vi "test_PhotonPoseEstimator_pnpDistanceTrigSolve.vi"(8 "error in (no error)":errorcluster) -> (0 "error out":errorcluster, 3 "Test Passed":bool)   [LabVIEW 2019]
uses:
  <vilib>/Rock Robotics/WPI/ThirdParty/PhotonVisionLib/TypeDef/PhotonEstimatedRobotPoseType.ctl
  <vilib>/Rock Robotics/WPI/ThirdParty/JAS_Junk/TrajLib/TypeDef/POSE3D.ctl
  <vilib>/Rock Robotics/WPI/ThirdParty/JAS_Junk/TrajLib/TypeDef/TRANSLATION3D.ctl
  <vilib>/Rock Robotics/WPI/ThirdParty/JAS_Junk/TrajLib/TypeDef/ROTATION3D.ctl
  <vilib>/Rock Robotics/WPI/ThirdParty/JAS_Junk/TrajLib/TypeDef/QUATERNION.ctl
  <vilib>/Rock Robotics/WPI/ThirdParty/PhotonVisionLib/TypeDef/PhotonTrackedTargetType.ctl
  <vilib>/Rock Robotics/WPI/ThirdParty/PhotonVisionLib/TypeDef/TargetCornerType.ctl
  <vilib>/Rock Robotics/WPI/ThirdParty/JAS_Junk/TrajLib/TypeDef/TRANSFORM3D.ctl
  <vilib>/Rock Robotics/WPI/ThirdParty/PhotonVisionLib/Enum/PhotonPoseStrategy_ENUM.ctl
  <vilib>/Rock Robotics/WPI/ThirdParty/JAS_Junk/TrajLib/VI/Quaternion_New_Default.vi
  <vilib>/Rock Robotics/WPI/ThirdParty/JAS_Junk/TrajLib/VI/Quaternion_New.vi
  <vilib>/Rock Robotics/WPI/ThirdParty/PhotonVisionLib/SubVI/PhotonTargetModel_New_AprilTag36H11.vi
  <vilib>/Rock Robotics/WPI/ThirdParty/JAS_Junk/TrajLib/VI/TimeInterpRotation2d_New.vi
  <vilib>/Rock Robotics/WPI/ThirdParty/JAS_Junk/TrajLib/VI/TimeInterpRotation2d_AddSample.vi
  <vilib>/Rock Robotics/WPI/ThirdParty/JAS_Junk/TrajLib/VI/Rotation3d_ToRotation2d.vi
  <vilib>/Rock Robotics/WPI/ThirdParty/PhotonVisionLib/SubVI/PhotonPoseEstimator_Update_All.vi
  <vilib>/Rock Robotics/WPI/ThirdParty/JAS_Junk/TrajLib/VI/Quaternion_Get_All.vi
  <vilib>/Rock Robotics/WPI/ThirdParty/JAS_Junk/TrajLib/VI/Rotation3d_GetQuaterion.vi
  <vilib>/Rock Robotics/WPI/ThirdParty/PhotonVisionLib/SubVI/PhotonPoseEstimator_GetEmptyPose.vi
  <vilib>/Rock Robotics/WPI/ThirdParty/PhotonVisionLib/SubVI/PhotonPoseEstimator_EstimatePnpDistanceTrigSolvePose.vi
  <vilib>/Rock Robotics/WPI/ThirdParty/PhotonVisionLib/SubVI/PhotonPoseEstimator_SetLastPose.vi
  <vilib>/Rock Robotics/WPI/ThirdParty/JAS_Junk/TrajLib/VI/Transform3d_Equals.vi
  <vilib>/Rock Robotics/WPI/ThirdParty/PhotonVisionLib/SubVI/PhotonPoseEstimator_SetCamera.vi
  <vilib>/Rock Robotics/WPI/ThirdParty/PhotonVisionLib/SubVI/PhotonPoseEstimator_SetRobotToCameraTransform.vi
  <vilib>/Rock Robotics/WPI/ThirdParty/PhotonVisionLib/SubVI/PhotonEstimatedRobotPose_GetAll.vi
  <vilib>/Rock Robotics/WPI/ThirdParty/JAS_Junk/TrajLib/VI/Pose3d_ToPose2d.vi
  <vilib>/Rock Robotics/WPI/ThirdParty/PhotonVisionLib/SubVI/PhotonTargetModel_New_RectPlanar.vi
  <vilib>/Rock Robotics/WPI/ThirdParty/JAS_Junk/TrajLib/VI/TimeInterpRotation2d_CleanUp.vi
  <vilib>/Rock Robotics/WPI/ThirdParty/JAS_Junk/TrajLib/Rotation2d_CreateAngle.vi
  <vilib>/Rock Robotics/WPI/ThirdParty/PhotonVisionLib/SubVI/PhotonPoseEstimator_EstimateLowestAmbiguityPose.vi
  <vilib>/Rock Robotics/WPI/ThirdParty/PhotonVisionLib/SubVI/PhotonPoseEstimator_EstimateClosestToCameraHeightPose.vi
  <vilib>/Rock Robotics/WPI/ThirdParty/PhotonVisionLib/SubVI/PhotonPoseEstimator_EstimateClosestToReferencePose.vi
  <vilib>/Rock Robotics/WPI/ThirdParty/PhotonVisionLib/SubVI/PhotonPoseEstimator_GetReferencePose.vi
  <vilib>/Rock Robotics/WPI/ThirdParty/PhotonVisionLib/SubVI/PhotonPoseEstimator_GetLastPose.vi
  <vilib>/Rock Robotics/WPI/ThirdParty/PhotonVisionLib/SubVI/PhotonPoseEstimator_SetReferencePose.vi
  <vilib>/Rock Robotics/WPI/ThirdParty/PhotonVisionLib/SubVI/PhotonPoseEstimator_EstimateClosestToLastPose.vi
  <vilib>/Rock Robotics/WPI/ThirdParty/PhotonVisionLib/SubVI/PhotonPoseEstimator_EstimateAverageBestTargetsPose.vi
  <vilib>/Rock Robotics/WPI/ThirdParty/PhotonVisionLib/SubVI/PhotonPoseEstimator_EstimateMultiTagOnCoprocPose.vi
  <vilib>/Rock Robotics/WPI/ThirdParty/PhotonVisionLib/SubVI/PhotonPoseEstimator_Strategy_constrainedPnpStrategy.vi
  <vilib>/Rock Robotics/WPI/ThirdParty/JAS_Junk/TrajLib/VI/Rotation3d_Create_AxisAngle.vi
  <vilib>/Rock Robotics/WPI/ThirdParty/JAS_Junk/TrajLib/VI/Pose3d_New.vi
  <vilib>/Rock Robotics/WPI/ThirdParty/PhotonVisionLib/SubVI/PhotonPipelineResult_HasTargets.vi
  <vilib>/Rock Robotics/WPI/ThirdParty/PhotonVisionLib/SubVI/PhotonPipelineResult_GetBestTarget.vi
  <vilib>/Rock Robotics/WPI/ThirdParty/PhotonVisionLib/SubVI/PhotonTrackedTarget_GetPoseAmbiguity.vi
  <vilib>/Rock Robotics/WPI/ThirdParty/PhotonVisionLib/SubVI/PhotonTrackedTarget_GetPitch.vi
  <vilib>/Rock Robotics/WPI/ThirdParty/PhotonVisionLib/SubVI/PhotonTrackedTarget_GetYaw.vi
  <vilib>/Rock Robotics/WPI/ThirdParty/JAS_Junk/TrajLib/Units_DegreesToRadians.vi
  <vilib>/Rock Robotics/WPI/ThirdParty/PhotonVisionLib/SubVI/PhotonTrackedTarget_GetBestCameraToTarget.vi
  <vilib>/Rock Robotics/WPI/ThirdParty/JAS_Junk/TrajLib/VI/Transform3d_GetTranslation3d.vi
  <vilib>/Rock Robotics/WPI/ThirdParty/JAS_Junk/TrajLib/VI/Translation3d_GetNorm.vi
  <vilib>/Rock Robotics/WPI/ThirdParty/JAS_Junk/TrajLib/VI/Translation3d_Create_DistAng.vi
  <vilib>/Rock Robotics/WPI/ThirdParty/JAS_Junk/TrajLib/VI/Translation3d_RotateBy.vi
  <vilib>/Rock Robotics/WPI/ThirdParty/JAS_Junk/TrajLib/VI/Translation3d_ToTranslation2d.vi
  <vilib>/Rock Robotics/WPI/ThirdParty/JAS_Junk/TrajLib/Translation2d_RotateBy.vi
  <vilib>/Rock Robotics/WPI/ThirdParty/JAS_Junk/TrajLib/VI/Transform3d_GetRotation3d.vi
  <vilib>/Rock Robotics/WPI/ThirdParty/JAS_Junk/TrajLib/Pose2d_getTranslation.vi
  <vilib>/Rock Robotics/WPI/ThirdParty/JAS_Junk/TrajLib/Translation2d_Plus.vi
  <vilib>/Rock Robotics/WPI/ThirdParty/JAS_Junk/TrajLib/Translation2d_UnaryMinus.vi
  <vilib>/Rock Robotics/WPI/ThirdParty/JAS_Junk/TrajLib/Pose2d_New_TRRO.vi
  <vilib>/Rock Robotics/WPI/ThirdParty/JAS_Junk/TrajLib/VI/Pose3d_New_Pose2d.vi
  <vilib>/Rock Robotics/WPI/ThirdParty/JAS_Junk/TrajLib/VI/TimeInterpRotation2d_GetSample.vi
  <vilib>/Rock Robotics/WPI/ThirdParty/PhotonVisionLib/SubVI/PhotonPoseEstimator_GetFieldTags.vi
  <vilib>/Rock Robotics/WPI/ThirdParty/PhotonVisionLib/SubVI/PhotonTrackedTarget_GetFiducialId.vi
  <vilib>/Rock Robotics/WPI/ThirdParty/JAS_Junk/TrajLib/VI/AprilTagFieldLayout_GetTagPose.vi
  <vilib>/Rock Robotics/WPI/ThirdParty/PhotonVisionLib/SubVI/PhotonPoseEstimator_GetHeadingBuffer.vi
  <vilib>/Rock Robotics/WPI/ThirdParty/PhotonVisionLib/SubVI/PhotonPoseEstimator_GetRobotToCameraTransform.vi
  <vilib>/Rock Robotics/WPI/ThirdParty/PhotonVisionLib/SubVI/PhotonPoseEstimator_GetHighestAmbiguity.vi
  <vilib>/Rock Robotics/WPI/ThirdParty/PhotonVisionLib/SubVI/PhotonEstimatedRobotPose_New.vi
  <vilib>/Rock Robotics/WPI/ThirdParty/PhotonVisionLib/SubVI/PhotonPipelineResult_GetTargets.vi
  <vilib>/Rock Robotics/WPI/ThirdParty/JAS_Junk/TrajLib/VI/Rotation3d_Equals.vi
  <vilib>/Rock Robotics/WPI/ThirdParty/JAS_Junk/TrajLib/VI/Translation3d_Equals.vi
  <vilib>/Rock Robotics/WPI/ThirdParty/JAS_Junk/TrajLib/VI/Pose3d_getTranslation3d.vi
  <vilib>/Rock Robotics/WPI/ThirdParty/JAS_Junk/TrajLib/VI/Pose3d_getRotation3d.vi
  <vilib>/Rock Robotics/WPI/ThirdParty/PhotonVisionLib/SubVI/PhotonTargetModel_New.vi
  <vilib>/Rock Robotics/WPI/ThirdParty/JAS_Junk/TrajLib/VI/Pose3d_TransformBy.vi
  <vilib>/Rock Robotics/WPI/ThirdParty/JAS_Junk/TrajLib/VI/Transform3d_Inverse.vi
  <vilib>/Rock Robotics/WPI/ThirdParty/PhotonVisionLib/SubVI/PhotonPoseEstimator_Strategy_closestToCameraHeight_calc.vi
  <vilib>/Rock Robotics/WPI/ThirdParty/PhotonVisionLib/SubVI/PhotonTrackedTarget_GetAltCameraToTarget.vi
  <vilib>/Rock Robotics/WPI/ThirdParty/PhotonVisionLib/SubVI/PhotonPoseEstimator_Strategy_closestToReferencePose_calc.vi
  <vilib>/Rock Robotics/WPI/ThirdParty/PhotonVisionLib/SubVI/PhotonPoseEstimator_Strategy_averageBestTargets_calc.vi
  <vilib>/Rock Robotics/WPI/ThirdParty/JAS_Junk/TrajLib/VI/Rotation3d_Plus.vi
  <vilib>/Rock Robotics/WPI/ThirdParty/JAS_Junk/TrajLib/VI/Translation3d_Plus.vi
  <vilib>/Rock Robotics/WPI/ThirdParty/JAS_Junk/TrajLib/VI/Translation3d_Times.vi
  <vilib>/Rock Robotics/WPI/ThirdParty/JAS_Junk/TrajLib/VI/Rotation3d_Times.vi
  <vilib>/Rock Robotics/WPI/ThirdParty/JAS_Junk/TrajLib/VI/Translation3d_Create_Default.vi
  <vilib>/Rock Robotics/WPI/ThirdParty/JAS_Junk/TrajLib/VI/Pose3d_New_Trans3dRot3d.vi
  <vilib>/Rock Robotics/WPI/ThirdParty/JAS_Junk/TrajLib/VI/Pose3d_New_Default.vi
  <vilib>/Rock Robotics/WPI/ThirdParty/JAS_Junk/TrajLib/VI/Pose3d_Plus.vi
  <vilib>/Rock Robotics/WPI/ThirdParty/JAS_Junk/TrajLib/VI/Pose3d_RelativeTo.vi
  <vilib>/Rock Robotics/WPI/ThirdParty/JAS_Junk/TrajLib/VI/AprilTagFieldLayout_GetOriginPosition.vi
  <vilib>/Rock Robotics/WPI/ThirdParty/PhotonVisionLib/SubVI/PhotonPipelineResult_GetMultiTagResult.vi
  <vilib>/Rock Robotics/WPI/ThirdParty/JAS_Junk/TrajLib/VI/Vector_Norm.vi
  <vilib>/Rock Robotics/WPI/ThirdParty/JAS_Junk/TrajLib/VecBuilder_ArrayBy1Fill.vi
  <vilib>/Rock Robotics/WPI/ThirdParty/JAS_Junk/TrajLib/Transform2d_Create_TransRot.vi
  <vilib>/Rock Robotics/WPI/ThirdParty/JAS_Junk/TrajLib/VI/Quaternion_Times.vi
  <vilib>/Rock Robotics/WPI/ThirdParty/JAS_Junk/TrajLib/VI/Quaternion_Inverse.vi
  <vilib>/Rock Robotics/WPI/ThirdParty/JAS_Junk/TrajLib/Translation2d_Create.vi
  <vilib>/Rock Robotics/WPI/ThirdParty/JAS_Junk/TrajLib/Pose2d_getXYAngle.vi
  <vilib>/Rock Robotics/WPI/ThirdParty/JAS_Junk/TrajLib/Rotation2d_Interpolate.vi
  <vilib>/Rock Robotics/WPI/ThirdParty/JAS_Junk/TrajLib/VI/AprilTag_GetAll.vi
  <vilib>/Rock Robotics/WPI/ThirdParty/JAS_Junk/TrajLib/VI/Quaternion_Equals.vi
  <vilib>/Rock Robotics/WPI/ThirdParty/JAS_Junk/TrajLib/VI/Rotation3d_UnaryMinus.vi
  <vilib>/Rock Robotics/WPI/ThirdParty/JAS_Junk/TrajLib/VI/Translation3d_UnaryMinus.vi
  <vilib>/Rock Robotics/WPI/ThirdParty/JAS_Junk/TrajLib/VI/Transform3d_GetXYZ.vi
  <vilib>/Rock Robotics/WPI/ThirdParty/JAS_Junk/TrajLib/VI/Pose3d_getXYZ.vi
  <vilib>/Rock Robotics/WPI/ThirdParty/PhotonVisionLib/SubVI/PhotonPoseEstimator_CalcDifference.vi
  <vilib>/Rock Robotics/WPI/ThirdParty/JAS_Junk/TrajLib/VI/Rotation3d_RotateBy.vi
  <vilib>/Rock Robotics/WPI/ThirdParty/JAS_Junk/TrajLib/VI/Translation3d_GetXYZ.vi
  <vilib>/Rock Robotics/WPI/ThirdParty/JAS_Junk/TrajLib/VI/Quaternion_Get_Vect.vi
  <vilib>/Rock Robotics/WPI/ThirdParty/JAS_Junk/TrajLib/VI/Quaternion_Get_W.vi
  <vilib>/Rock Robotics/WPI/ThirdParty/JAS_Junk/TrajLib/VI/Transform3d_Create_Pose3dPose3d.vi
  <vilib>/Rock Robotics/WPI/ThirdParty/JAS_Junk/TrajLib/MatBuilder_Create.vi
  <vilib>/Rock Robotics/WPI/ThirdParty/JAS_Junk/TrajLib/Rotation2d_Plus.vi
  <vilib>/Rock Robotics/WPI/ThirdParty/JAS_Junk/TrajLib/Rotation2d_Minus.vi
  <vilib>/Rock Robotics/WPI/ThirdParty/JAS_Junk/TrajLib/MathUtil_Clamp.vi
  <vilib>/Rock Robotics/WPI/ThirdParty/JAS_Junk/TrajLib/Rotation2d_Times.vi
  <vilib>/Rock Robotics/WPI/ThirdParty/JAS_Junk/TrajLib/VI/Rotation3d_Create_Quaternion.vi
  <vilib>/Rock Robotics/WPI/ThirdParty/JAS_Junk/TrajLib/VI/Translation3d_GetDistance.vi
  <vilib>/Rock Robotics/WPI/ThirdParty/JAS_Junk/TrajLib/VI/Translation3d_Minus.vi
  <vilib>/Rock Robotics/WPI/ThirdParty/JAS_Junk/TrajLib/VI/Rotation3d_Minus.vi
  <vilib>/Rock Robotics/WPI/ThirdParty/JAS_Junk/TrajLib/Rotation2d_RotateBy.vi
  <vilib>/Rock Robotics/WPI/ThirdParty/JAS_Junk/TrajLib/Rotation2d_UnaryMinus.vi
  <vilib>/Rock Robotics/WPI/ThirdParty/JAS_Junk/TrajLib/VI/Quaternion_Normalize.vi
  <vilib>/Rock Robotics/WPI/ThirdParty/JAS_Junk/TrajLib/Rotation2d_CreateXY.vi
  <vilib>/Rock Robotics/WPI/ThirdParty/JAS_Junk/TrajLib/Util_CalcDist.vi
  <vilib>/Rock Robotics/WPI/ThirdParty/PhotonVisionLib/SubVI/PhotonVision_Globals.vi
  <vilib>/gmath/interp.llb/Search Ordered Table.vi
  <vilib>/Rock Robotics/WPI/ThirdParty/JAS_Junk/TrajLib/Trajectory_Library.lvlib
  <vilib>/Rock Robotics/WPI/ThirdParty/PhotonVisionLib/PhotonVisionLib.lvlib
  <vilib>/Rock Robotics/WPI/ThirdParty/JAS_Junk/TrajLib/TypeDef/AprilTag.ctl
  <vilib>/Rock Robotics/WPI/ThirdParty/JAS_Junk/TrajLib/Enum/AprilTagFieldLayoutOrignPosition_ENUM.ctl
  <vilib>/Rock Robotics/WPI/ThirdParty/JAS_Junk/TrajLib/TypeDef/AprilTagFieldLayout.ctl
  <vilib>/Rock Robotics/WPI/ThirdParty/PhotonVisionLib/TypeDef/PhotonTargetModel.ctl
  <vilib>/Rock Robotics/WPI/ThirdParty/PhotonVisionLib/TypeDef/PhotonPoseEstimatorType.ctl
panel:
  out "out PhotonPoseEstimator":T1={"LastPose"={"Translation3d"={"X"=0.0, "Y"=0.0, "Z"=0.0}, "Rotation3d"={"Q_quaternion"={"R"=1.0, "V"=[0.0, 0.0, 0.0]}}}, "ReferencePose"={"Translation3d"={"X"=0.0, "Y"=0.0, "Z"=0.0}, "Rotation3d"={"Q_quaternion"={"R"=1.0, "V"=[0.0, 0.0, 0.0]}}}, "FieldTags"={"AprilTagMap"={}, "FieldLength"=0.0, "FieldWidth"=0.0, "OriginPosition "=enum."kBlueAllianceWallRightSide,", "OriginPose3d"={"Translation3d"={"X"=0.0, "Y"=0.0, "Z"=0.0}, "Rotation3d"={"Q_quaternion"={"R"=1.0, "V"=[0.0, 0.0, 0.0]}}}}, "PrimaryStratety"=enum."LOWEST_AMBIGUITY", "Camera"="", "RobotToCamera"={"TRANSLATION3D"={"X"=0.0, "Y"=0.0, "Z"=0.0}, "ROTATION3D"={"Q_quaternion"={"R"=1.0, "V"=[0.0, 0.0, 0.0]}}, "XF"=FALSE}, "ReportedErrors"=[], "HighestAmbiguity"=10.0, "MultiTagFallbackStrategy"=enum."LOWEST_AMBIGUITY", "PoseCacheTimeoutSec"=-1.0, "PhotonTargetModel"={"Vertices"=[], "IsPlaner"=FALSE, "IsSpherical"=FALSE}, "BaseNTName"="/photonvision"} {"PhotonTargetModel"."Vertices"."Z" format="%14.3f"; "PhotonTargetModel"."Vertices"."Y" format="%14.3f"; "PhotonTargetModel"."Vertices"."X" format="%14.3f"; "RobotToCamera"."TRANSLATION3D"."Z" format="%14.3f"; "RobotToCamera"."TRANSLATION3D"."Y" format="%14.3f"; "RobotToCamera"."TRANSLATION3D"."X" format="%14.3f"; "FieldTags"."OriginPose3d"."Translation3d"."Z" format="%14.3f"; "FieldTags"."OriginPose3d"."Translation3d"."Y" format="%14.3f"; "FieldTags"."OriginPose3d"."Translation3d"."X" format="%14.3f"; "ReferencePose"."Translation3d"."Z" format="%14.3f"; "ReferencePose"."Translation3d"."Y" format="%14.3f"; "ReferencePose"."Translation3d"."X" format="%14.3f"; "LastPose"."Translation3d"."Z" format="%14.3f"; "LastPose"."Translation3d"."Y" format="%14.3f"; "LastPose"."Translation3d"."X" format="%14.3f"}
  out "Test 2 Passed":bool
  out "Test 1 Passed":bool
  out "Pos Found":bool
  out "PhotonEstimatedRobotPose":T12={"EstimatedPose"={"Translation3d"={"X"=0.0, "Y"=0.0, "Z"=0.0}, "Rotation3d"={"Q_quaternion"={"R"=1.0, "V"=[0.0, 0.0, 0.0]}}}, "TimeStamp_Seconds"=0.0, "targetsUsed"=[], "Strategy"=enum."LOWEST_AMBIGUITY"} {"targetsUsed"."AltCameraToTarget"."TRANSLATION3D"."Z" format="%14.3f"; "targetsUsed"."AltCameraToTarget"."TRANSLATION3D"."Y" format="%14.3f"; "targetsUsed"."AltCameraToTarget"."TRANSLATION3D"."X" format="%14.3f"; "targetsUsed"."BestCameraToTarget"."TRANSLATION3D"."Z" format="%14.3f"; "targetsUsed"."BestCameraToTarget"."TRANSLATION3D"."Y" format="%14.3f"; "targetsUsed"."BestCameraToTarget"."TRANSLATION3D"."X" format="%14.3f"; "EstimatedPose"."Translation3d"."Z" format="%14.3f"; "EstimatedPose"."Translation3d"."Y" format="%14.3f"; "EstimatedPose"."Translation3d"."X" format="%14.3f"}
  out "Test 0 Passed":bool
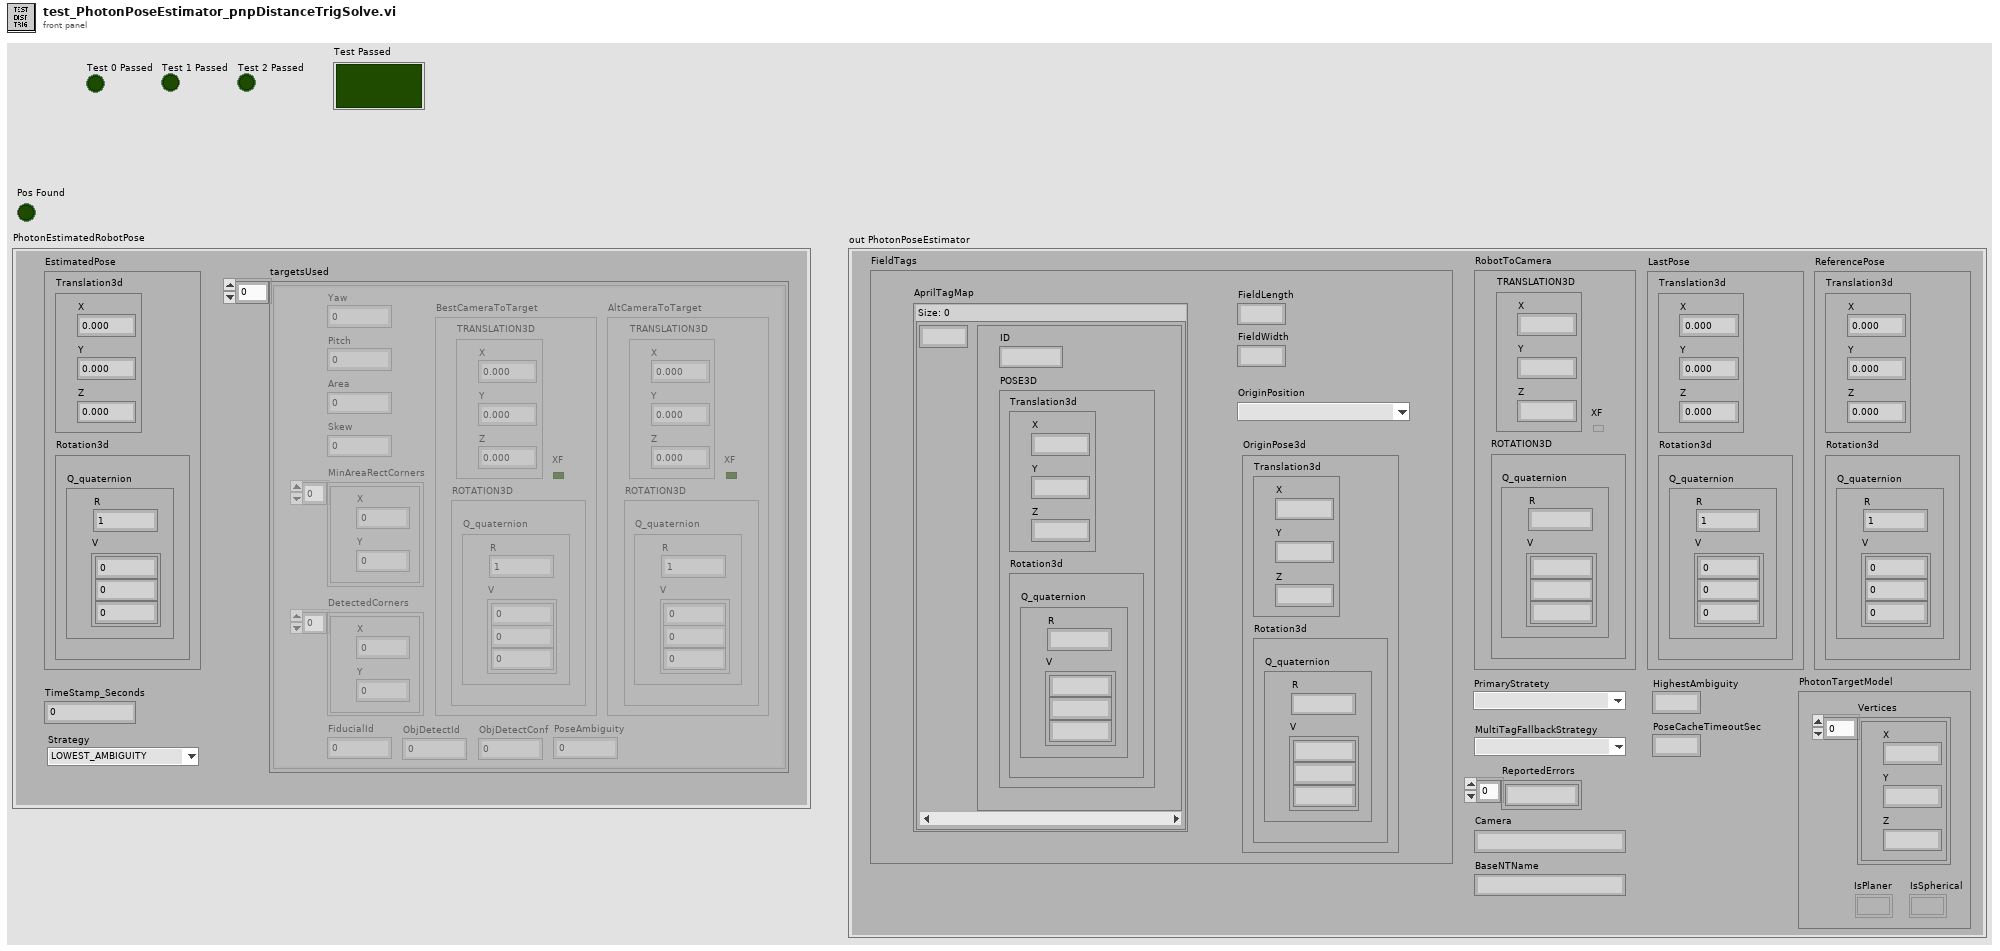
[diagram p1: front panel]
types:
  T1 = typedef "PhotonVisionLib.lvlib/PhotonPoseEstimatorType.ctl" = cluster{"LastPose":T2, "ReferencePose":T2, "FieldTags":T6, "PrimaryStratety":T9, "Camera":string, "RobotToCamera":T10, "ReportedErrors":dbl[], "HighestAmbiguity":dbl, "MultiTagFallbackStrategy":T9, "PoseCacheTimeoutSec":dbl, "PhotonTargetModel":T11, "BaseNTName":string}
  T2 = typedef "Trajectory_Library.lvlib/POSE3D.ctl" = cluster{"Translation3d":T3, "Rotation3d":T4}
  T3 = typedef "Trajectory_Library.lvlib/TRANSLATION3D.ctl" = cluster{"X":dbl, "Y":dbl, "Z":dbl}
  T4 = typedef "Trajectory_Library.lvlib/ROTATION3D.ctl" = cluster{"Q_quaternion":T5}
  T5 = typedef "Trajectory_Library.lvlib/QUATERNION.ctl" = cluster{"R":dbl, "V":dbl[]}
  T6 = typedef "Trajectory_Library.lvlib/AprilTagFieldLayout.ctl" = cluster{"AprilTagMap":map{i32, T7}, "FieldLength":dbl, "FieldWidth":dbl, "OriginPosition ":T8, "OriginPose3d":T2}
  T7 = typedef "Trajectory_Library.lvlib/AprilTag.ctl" = cluster{"ID":i32, "POSE3D":T2}
  T8 = typedef "Trajectory_Library.lvlib/AprilTagFieldLayoutOrignPosition_ENUM.ctl" = enum16{"kBlueAllianceWallRightSide,", "kRedAllianceWallRightSide,"}
  T9 = typedef "PhotonVisionLib.lvlib/PhotonPoseStrategy_ENUM.ctl" = enum16{"LOWEST_AMBIGUITY", "CLOSEST_TO_CAMERA_HEIGHT", "CLOSEST_TO_REFERENCE_POSE", "CLOSEST_TO_LAST_POSE", "AVERAGE_BEST_TARGETS", "MULTI_TAG_PNP_ON_COPROCESSOR", "MULTI_TAG_PNP_ON_RIO", "PNP_DISTANCE_TRIG_SOLVE", "CONSTRAINED_SOLVEPNP"}
  T10 = typedef "Trajectory_Library.lvlib/TRANSFORM3D.ctl" = cluster{"TRANSLATION3D":T3, "ROTATION3D":T4, "XF":bool}
  T11 = typedef "PhotonVisionLib.lvlib/PhotonTargetModel.ctl" = cluster{"Vertices":T3[], "IsPlaner":bool, "IsSpherical":bool}
  T12 = typedef "PhotonVisionLib.lvlib/PhotonEstimatedRobotPoseType.ctl" = cluster{"EstimatedPose":T2, "TimeStamp_Seconds":dbl, "targetsUsed":T13[], "Strategy":T9}
  T13 = typedef "PhotonVisionLib.lvlib/PhotonTrackedTargetType.ctl" = cluster{"Yaw":dbl, "Pitch":dbl, "Area":dbl, "Skew":dbl, "MinAreaRectCorners":T14[], "BestCameraToTarget":T10, "FiducialId":i32, "AltCameraToTarget":T10, "PoseAmbiguity":dbl, "DetectedCorners":T14[], "ObjDetectId":i32, "ObjDetectConf":sgl}
  T14 = typedef "PhotonVisionLib.lvlib/TargetCornerType.ctl" = cluster{"X":dbl, "Y":dbl}
  T15 = typedef "PhotonVisionLib.lvlib/PhotonPipelineMetadataType.ctl" = cluster{"CaptureTimestampMicros":i64, "PublishTimestampMicros":i64, "SequenceID":i64, "TimeSinceLastPong":i64}
  T16 = typedef "PhotonVisionLib.lvlib/PhotonPipelineResultType.ctl" = cluster{"Targets":T13[], "PhotonMultiTargetPNPResult":T17, "PhotonPipelineMetadata":T15}
  T17 = typedef "PhotonVisionLib.lvlib/PhotonMultiTargetPNPResultType.ctl" = cluster{"PhotonPNPResult":T18, "FiducialIDsUsed":i16[]}
  T18 = typedef "PhotonVisionLib.lvlib/PhotonPNPResultType.ctl" = cluster{"IsPresent":bool, "bestReprojErr":dbl, "altReprojErr":dbl, "ambiguity":dbl, "Best":T10, "Alt":T10}
  T19 = typedef "PhotonVisionLib.lvlib/PhotonPoseEstimator_Configuration.ctl" = cluster{"Primary Strategy":T9, "Camera":string, "Initial Pose":T2, "HighestAmbiguity":dbl, "RobotToCamera":T10, "FallBack Strategy":T9, "BaseNTName":string}
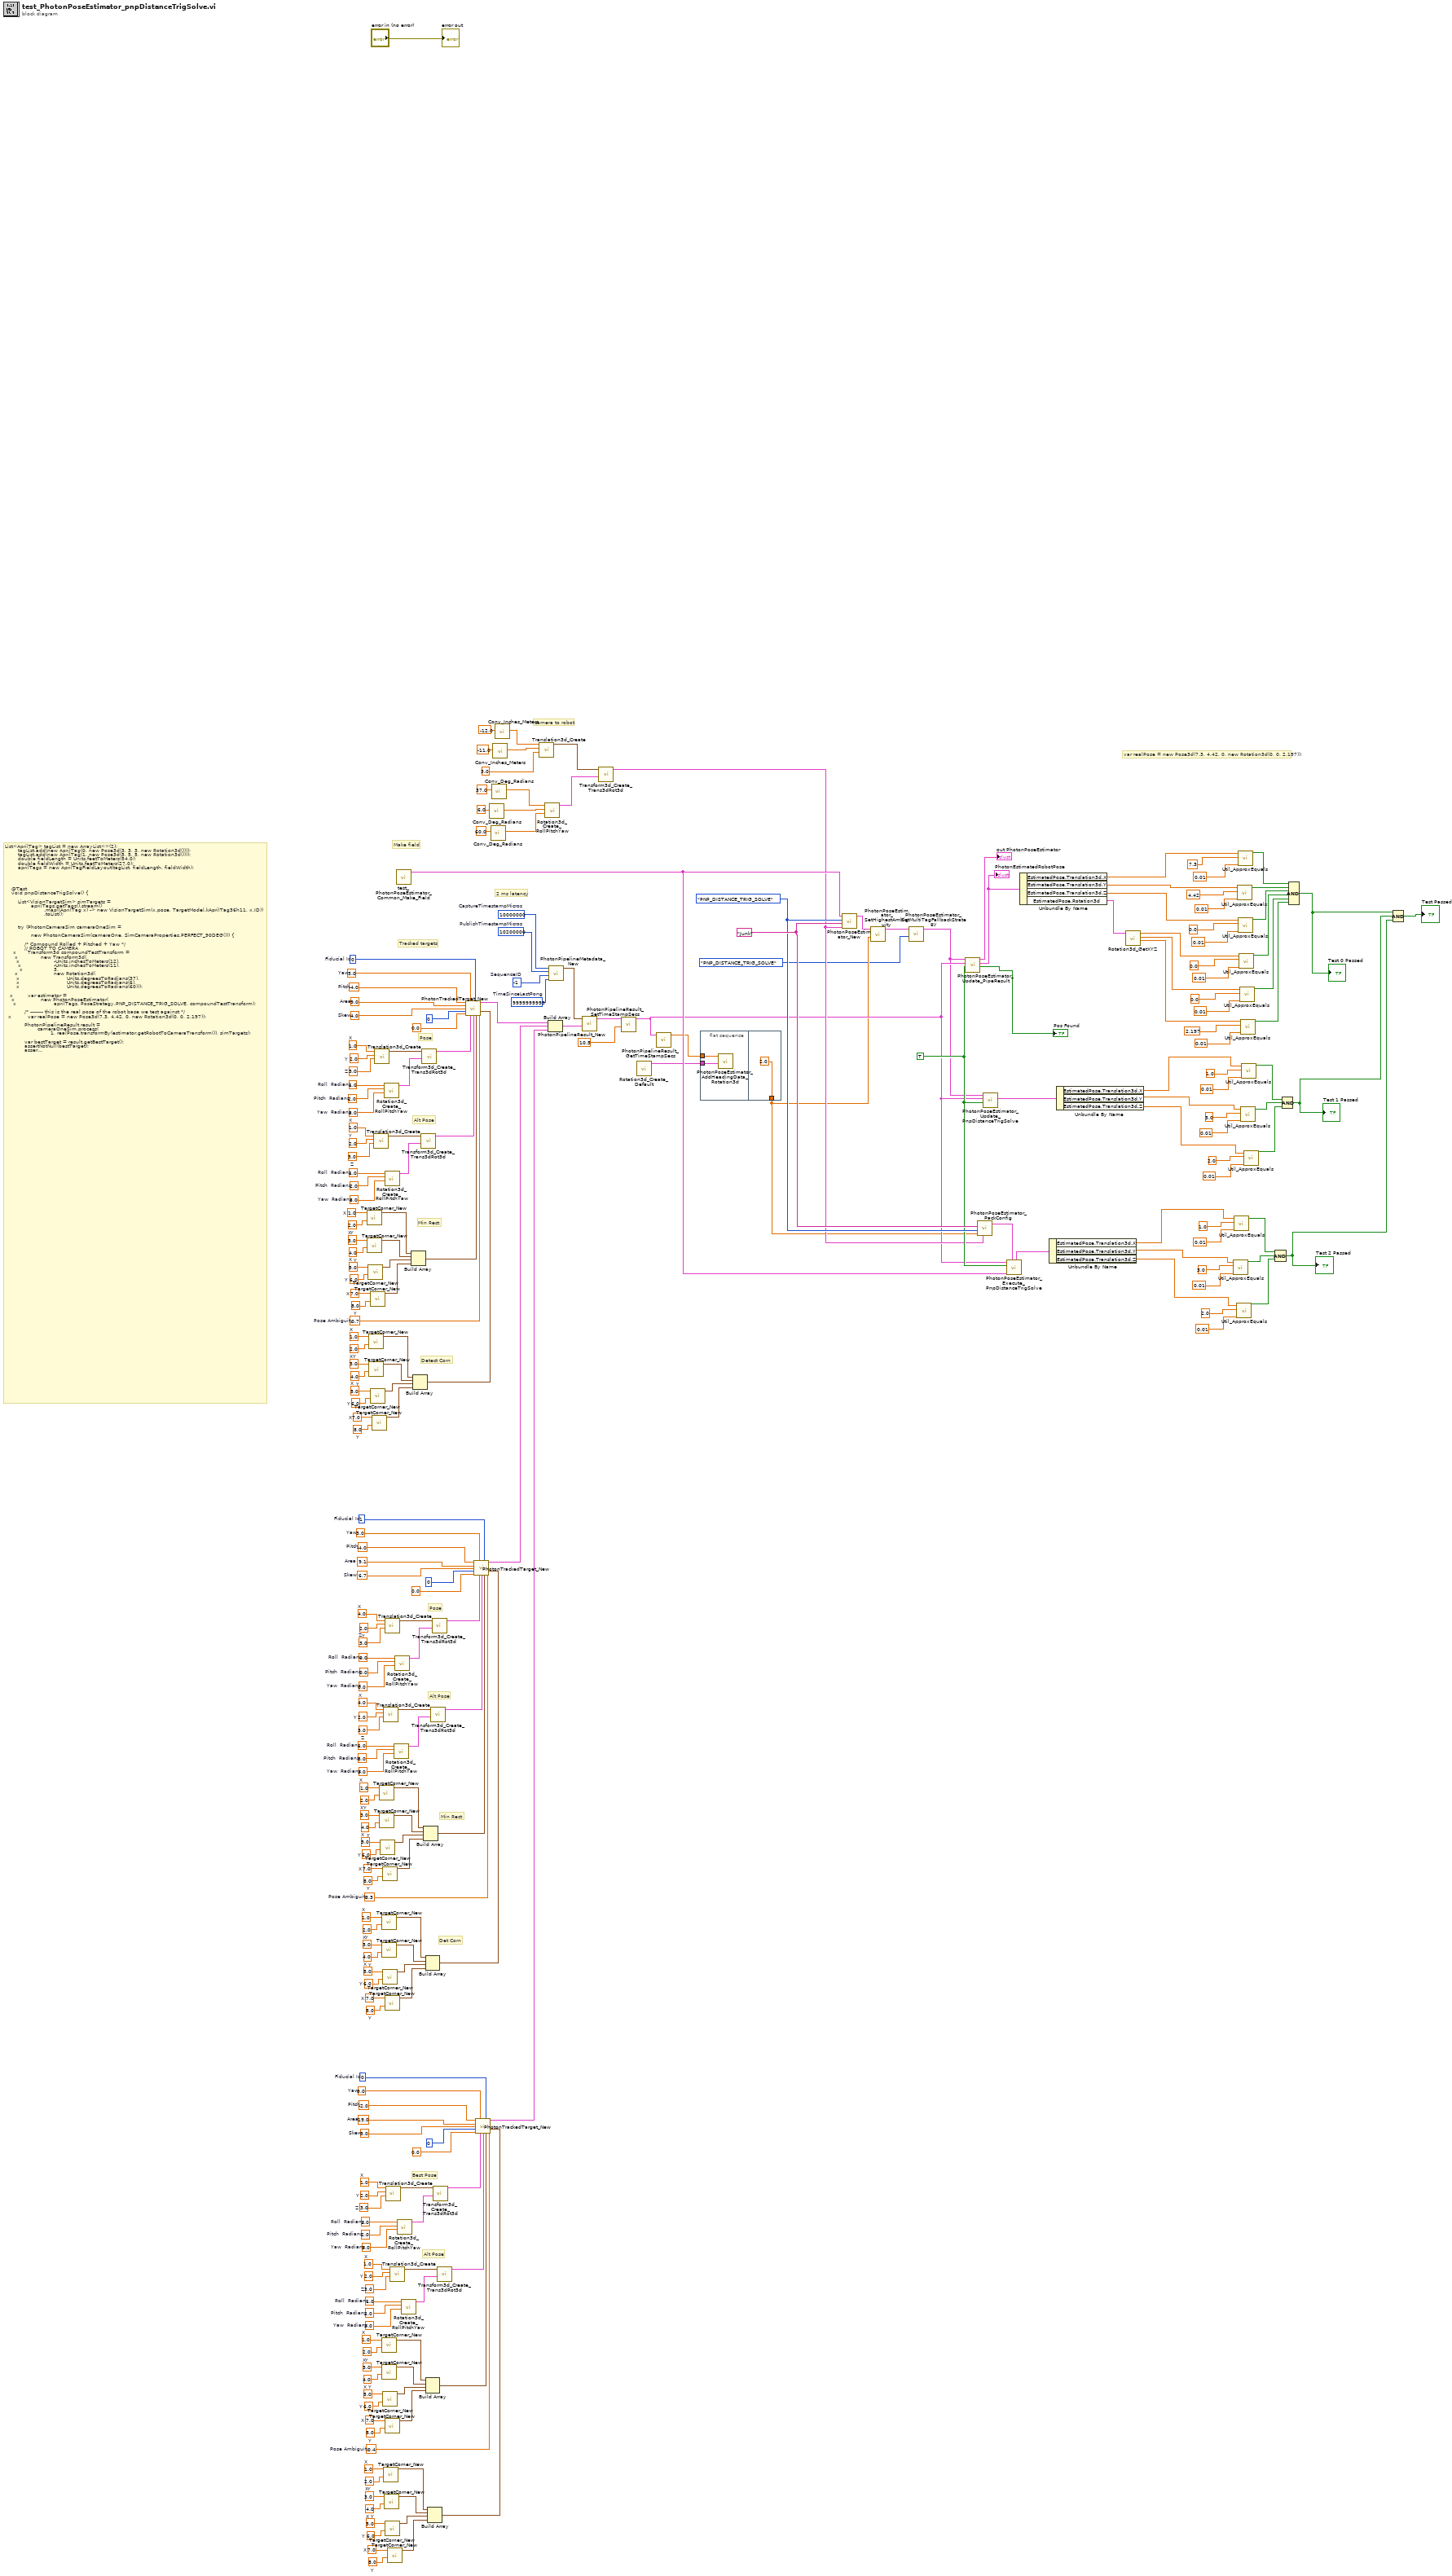
[diagram p0: block diagram]
diagram:
  w77 = i64 10000000  # CaptureTimestampMicros
  w78 = i64 10200000  # PublishTimestampMicros
  w79 = i64 -1  # SequenceID
  w80 = i64 9999999999  # TimeSinceLastPong
  w37 = TRUE ("Has Results")
  w42 = "Junk" ("Camera")
  w41 = PhotonPoseStrategy_ENUM."PNP_DISTANCE_TRIG_SOLVE" ("Strategy")
  w104 = 1.0  # Roll  Radians
  w103 = 2.0  # Pitch  Radians
  w102 = 3.0  # Yaw  Radians
  w107 = 3.0  # Z
  w106 = 1.0  # X
  w105 = 2.0  # Y
  w112 = 1.0  # Roll  Radians
  w111 = 2.0  # Pitch  Radians
  w110 = 3.0  # Yaw  Radians
  w115 = 3.0  # Z
  w114 = 1.0  # X
  w113 = 2.0  # Y
  w122 = 7.0  # X
  w123 = 8.0  # Y
  w124 = 5.0  # X
  w125 = 6.0  # Y
  w126 = 3.0  # X
  w127 = 4.0  # Y
  w128 = 1.0  # X
  w129 = 2.0  # Y
  w134 = 7.0  # X
  w135 = 8.0  # Y
  w136 = 5.0  # X
  w137 = 6.0  # Y
  w138 = 3.0  # X
  w139 = 4.0  # Y
  w140 = 1.0  # X
  w141 = 2.0  # Y
  w142 = -2.0  # Pitch
  w143 = 19.0  # Area
  w144 = 3.0  # Skew
  w145 = 0  # Fiducial Id
  w146 = 0.4  # Pose Ambiguity
  w147 = 9.0  # Yaw
  w154 = 0.0  # Roll  Radians
  w153 = 0.0  # Pitch  Radians
  w152 = 0.0  # Yaw  Radians
  w157 = 3.0  # Z
  w156 = 4.0  # X
  w155 = 2.0  # Y
  w162 = 1.0  # Roll  Radians
  w161 = 5.0  # Pitch  Radians
  w160 = 3.0  # Yaw  Radians
  w165 = 3.0  # Z
  w164 = 4.0  # X
  w163 = 2.0  # Y
  w172 = 7.0  # X
  w173 = 8.0  # Y
  w174 = 5.0  # X
  w175 = 6.0  # Y
  w176 = 3.0  # X
  w177 = 4.0  # Y
  w178 = 1.0  # X
  w179 = 2.0  # Y
  w184 = 7.0  # X
  w185 = 8.0  # Y
  w186 = 5.0  # X
  w187 = 6.0  # Y
  w188 = 3.0  # X
  w189 = 4.0  # Y
  w190 = 1.0  # X
  w191 = 2.0  # Y
  w192 = -4.0  # Pitch
  w193 = 9.1  # Area
  w194 = 6.7  # Skew
  w195 = 1  # Fiducial Id
  w196 = 0.3  # Pose Ambiguity
  w197 = 3.0  # Yaw
  w204 = 1.0  # Roll  Radians
  w203 = 2.0  # Pitch  Radians
  w202 = 3.0  # Yaw  Radians
  w207 = 3.0  # Z
  w206 = 1.0  # X
  w205 = 2.0  # Y
  w212 = 1.0  # Roll  Radians
  w211 = 2.0  # Pitch  Radians
  w210 = 3.0  # Yaw  Radians
  w215 = 3.0  # Z
  w214 = 1.0  # X
  w213 = 2.0  # Y
  w222 = 7.0  # X
  w223 = 8.0  # Y
  w224 = 5.0  # X
  w225 = 6.0  # Y
  w226 = 3.0  # X
  w227 = 4.0  # Y
  w228 = 1.0  # X
  w229 = 2.0  # Y
  w234 = 7.0  # X
  w235 = 8.0  # Y
  w236 = 5.0  # X
  w237 = 6.0  # Y
  w238 = 3.0  # X
  w239 = 4.0  # Y
  w240 = 1.0  # X
  w241 = 2.0  # Y
  w242 = -4.0  # Pitch
  w243 = 9.0  # Area
  w244 = 4.0  # Skew
  w245 = 0  # Fiducial Id
  w246 = 0.7  # Pose Ambiguity
  w247 = 3.0  # Yaw
  # "var realPose = new Pose3d(7.3, 4.42, 0, new Rotation3d(0, 0, 2.197));"
  # "camera to robot"
  # "List<AprilTag> tagList = new ArrayList<>(2);\n        tagList.add(new AprilTag(0, new Pose3d(3, 3, 3, new Rotation3d())));\n        tagList.add(new AprilTag(1, new Pose3d(5, 5, 5, new Rotation3d())));\n        double fieldLength = Units.feetToMeters(54.0);\n        double fieldWidth = Units.feetToMeters(27.0);\n        aprilTags = new AprilTagFieldLayout(tagList, fieldLength, fieldWidth);\n\n\n\n\n    @Test\n    void pnpDistanceTrigSolve() {\n\n        List<VisionTargetSim> simTargets =\n                aprilTags.getTags().stream()\n                        .map((AprilTag x) -> new VisionTargetSim(x.pose, TargetModel.kAprilTag36h11, x.ID))\n                        .toList();\n\n\n        try (PhotonCameraSim cameraOneSim =\n\n                new PhotonCameraSim(cameraOne, SimCameraProperties.PERFECT_90DEG())) {\n\n            /* Compound Rolled + Pitched + Yaw */\n          \t\t// ROBOT TO CAMERA\n     x       Transform3d compoundTestTransform =\n      x              new Transform3d(\n       x                     -Units.inchesToMeters(12),\n        x                    -Units.inchesToMeters(11),\n         x                   3,\n      x                      new Rotation3d(\n       x                             Units.degreesToRadians(37),\n       x                             Units.degreesToRadians(6),\n       x                             Units.degreesToRadians(60)));\n\n   x         var estimator =\n    x                new PhotonPoseEstimator(\n     x                       aprilTags, PoseStrategy.PNP_DISTANCE_TRIG_SOLVE, compoundTestTransform);\n\n            /* -------- this is the real pose of the robot base we test against */\n  x          var realPose = new Pose3d(7.3, 4.42, 0, new Rotation3d(0, 0, 2.197));\n\n            PhotonPipelineResult result =\n                    cameraOneSim.process(\n                            1, realPose.transformBy(estimator.getRobotToCameraTransform()), simTargets);\n\n            var bestTarget = result.getBestTarget();\n            assertNotNull(bestTarget);\n            assertEquals(0, bestTarget.fiducialId);\n\n            estimator.addHeadingData(result.getTimestampSeconds(), realPose.getRotation().toRotation2d());\n            var estimatedPose = estimator.update(result);\n\n            var pose = estimatedPose.get().estimatedPose;\n            assertEquals(realPose.getX(), pose.getX(), .01);\n            assertEquals(realPose.getY(), pose.getY(), .01);\n            assertEquals(0.0, pose.getZ(), .01);\n\n            /* -------- Straight on */\n            Transform3d straightOnTestTransform = new Transform3d(0, 0, 3, Rotation3d.kZero);\n\n            estimator.setRobotToCameraTransform(straightOnTestTransform);\n\n            /* Pose to compare with */\n            realPose = new Pose3d(4.81, 2.38, 0, new Rotation3d(0, 0, 2.818));\n            result =\n                    cameraOneSim.process(\n                            1, realPose.transformBy(estimator.getRobotToCameraTransform()), simTargets);\n\n            estimator.addHeadingData(result.getTimestampSeconds(), realPose.getRotation().toRotation2d());\n            estimatedPose = estimator.update(result);\n\n            pose = estimatedPose.get().estimatedPose;\n            assertEquals(realPose.getX(), pose.getX(), .01);\n            assertEquals(realPose.getY(), pose.getY(), .01);\n            assertEquals(0.0, pose.getZ(), .01);\n        }\n    }"
  # "2 ms latency"
  # "Det Corn"
  # "Min Rect"
  # "Pose"
  # "Detect Corn"
  # "Min Rect"
  # "Tracked targets"
  # "Make field"
  # "Best Pose"
  # "Alt Pose"
  # "Alt Pose"
  # "Pose"
  # "Alt Pose"
  n1 = call <vilib>:"TargetCorner_New.vi"("Y"=w241, "X"=w240) -> ("TargetCorner"=w233:T14)  [unwired: 9 in]
  n2 = call <vilib>:"TargetCorner_New.vi"("Y"=w239, "X"=w238) -> ("TargetCorner"=w232:T14)  [unwired: 9 in]
  n3 = call <vilib>:"TargetCorner_New.vi"("Y"=w237, "X"=w236) -> ("TargetCorner"=w231:T14)  [unwired: 9 in]
  n4 = call <vilib>:"TargetCorner_New.vi"("Y"=w229, "X"=w228) -> ("TargetCorner"=w221:T14)  [unwired: 9 in]
  n5 = call <vilib>:"TargetCorner_New.vi"("Y"=w227, "X"=w226) -> ("TargetCorner"=w220:T14)  [unwired: 9 in]
  n6 = call <vilib>:"TargetCorner_New.vi"("Y"=w235, "X"=w234) -> ("TargetCorner"=w230:T14)  [unwired: 9 in]
  n7 = call <vilib>:"TargetCorner_New.vi"("Y"=w225, "X"=w224) -> ("TargetCorner"=w219:T14)  [unwired: 9 in]
  n8 = call <vilib>:"TargetCorner_New.vi"("Y"=w223, "X"=w222) -> ("TargetCorner"=w218:T14)  [unwired: 9 in]
  n9 = call <vilib>:"Translation3d_Create.vi"("Z"=w215, "Y"=w213, "X"=w214) -> ("TRANSLATION3D"=w209:T3)  [unwired: 8 in]
  n10 = call <vilib>:"Translation3d_Create.vi"("Z"=w207, "Y"=w205, "X"=w206) -> ("TRANSLATION3D"=w201:T3)  [unwired: 8 in]
  n11 = call <vilib>:"TargetCorner_New.vi"("Y"=w191, "X"=w190) -> ("TargetCorner"=w183:T14)  [unwired: 9 in]
  n12 = call <vilib>:"TargetCorner_New.vi"("Y"=w189, "X"=w188) -> ("TargetCorner"=w182:T14)  [unwired: 9 in]
  n13 = call <vilib>:"TargetCorner_New.vi"("Y"=w187, "X"=w186) -> ("TargetCorner"=w181:T14)  [unwired: 9 in]
  n14 = call <vilib>:"TargetCorner_New.vi"("Y"=w179, "X"=w178) -> ("TargetCorner"=w171:T14)  [unwired: 9 in]
  n15 = call <vilib>:"TargetCorner_New.vi"("Y"=w141, "X"=w140) -> ("TargetCorner"=w133:T14)  [unwired: 9 in]
  n16 = call <vilib>:"TargetCorner_New.vi"("Y"=w177, "X"=w176) -> ("TargetCorner"=w170:T14)  [unwired: 9 in]
  n17 = call <vilib>:"TargetCorner_New.vi"("Y"=w139, "X"=w138) -> ("TargetCorner"=w132:T14)  [unwired: 9 in]
  n18 = call <vilib>:"TargetCorner_New.vi"("Y"=w185, "X"=w184) -> ("TargetCorner"=w180:T14)  [unwired: 9 in]
  n19 = call <vilib>:"TargetCorner_New.vi"("Y"=w175, "X"=w174) -> ("TargetCorner"=w169:T14)  [unwired: 9 in]
  n20 = call <vilib>:"TargetCorner_New.vi"("Y"=w137, "X"=w136) -> ("TargetCorner"=w131:T14)  [unwired: 9 in]
  n21 = call <vilib>:"Translation3d_Create.vi"("Z"=w165, "Y"=w163, "X"=w164) -> ("TRANSLATION3D"=w159:T3)  [unwired: 8 in]
  n22 = call <vilib>:"TargetCorner_New.vi"("Y"=w129, "X"=w128) -> ("TargetCorner"=w121:T14)  [unwired: 9 in]
  n23 = call <vilib>:"Rotation3d_Create_RollPitchYaw.vi"("Yaw"=w202, "Pitch"=w203, "Roll"=w204) -> ("Rotation3d"=w200:T4)  [unwired: 8 in]
  n24 = call <vilib>:"TargetCorner_New.vi"("Y"=w127, "X"=w126) -> ("TargetCorner"=w120:T14)  [unwired: 9 in]
  n25 = call <vilib>:"Rotation3d_Create_RollPitchYaw.vi"("Yaw"=w210, "Pitch"=w211, "Roll"=w212) -> ("Rotation3d"=w208:T4)  [unwired: 8 in]
  n26 = call <vilib>:"Translation3d_Create.vi"("Z"=w157, "Y"=w155, "X"=w156) -> ("TRANSLATION3D"=w151:T3)  [unwired: 8 in]
  n27 = call <vilib>:"TargetCorner_New.vi"("Y"=w173, "X"=w172) -> ("TargetCorner"=w168:T14)  [unwired: 9 in]
  n28 = call <vilib>:"TargetCorner_New.vi"("Y"=w135, "X"=w134) -> ("TargetCorner"=w130:T14)  [unwired: 9 in]
  n29 = call <vilib>:"TargetCorner_New.vi"("Y"=w125, "X"=w124) -> ("TargetCorner"=w119:T14)  [unwired: 9 in]
  n30 = call <vilib>:"Translation3d_Create.vi"("Z"=w107, "Y"=w105, "X"=w106) -> ("TRANSLATION3D"=w101:T3)  [unwired: 8 in]
  n31 = call <vilib>:"TargetCorner_New.vi"("Y"=w123, "X"=w122) -> ("TargetCorner"=w118:T14)  [unwired: 9 in]
  n32 = call <vilib>:"Translation3d_Create.vi"("Z"=w115, "Y"=w113, "X"=w114) -> ("TRANSLATION3D"=w109:T3)  [unwired: 8 in]
  n33 = call <vilib>:"Rotation3d_Create_RollPitchYaw.vi"("Yaw"=w160, "Pitch"=w161, "Roll"=w162) -> ("Rotation3d"=w158:T4)  [unwired: 8 in]
  n34 = call <vilib>:"Rotation3d_Create_RollPitchYaw.vi"("Yaw"=w152, "Pitch"=w153, "Roll"=w154) -> ("Rotation3d"=w150:T4)  [unwired: 8 in]
  n35 = call "test_PhotonPoseEstimator_Common_Make_Field.vi"() -> ("AprilTagFieldLayout"=w36:T6)  [unwired: 11 in]
  n36 = call <vilib>:"Rotation3d_Create_RollPitchYaw.vi"("Yaw"=w102, "Pitch"=w103, "Roll"=w104) -> ("Rotation3d"=w100:T4)  [unwired: 8 in]
  n37 = call <vilib>:"Rotation3d_Create_RollPitchYaw.vi"("Yaw"=w110, "Pitch"=w111, "Roll"=w112) -> ("Rotation3d"=w108:T4)  [unwired: 8 in]
  n38 = Build Array(w233, w232, w231, w230) -> (w217:T14[])
  n39 = Build Array(w221, w220, w219, w218) -> (w216:T14[])
  n40 = call <vilib>:"Transform3d_Create_Trans3dRot3d.vi"("Rotation3d"=w208, "Translation3d"=w209) -> ("Transform3d"=w198:T10)  [unwired: 9 in]
  n41 = call <vilib>:"Transform3d_Create_Trans3dRot3d.vi"("Rotation3d"=w200, "Translation3d"=w201) -> ("Transform3d"=w199:T10)  [unwired: 9 in]
  n42 = Build Array(w183, w182, w181, w180) -> (w167:T14[])
  n43 = Build Array(w171, w170, w169, w168) -> (w166:T14[])
  n44 = Build Array(w133, w132, w131, w130) -> (w117:T14[])
  n45 = Build Array(w121, w120, w119, w118) -> (w116:T14[])
  n46 = call <vilib>:"Transform3d_Create_Trans3dRot3d.vi"("Rotation3d"=w158, "Translation3d"=w159) -> ("Transform3d"=w148:T10)  [unwired: 9 in]
  n47 = call <vilib>:"Transform3d_Create_Trans3dRot3d.vi"("Rotation3d"=w150, "Translation3d"=w151) -> ("Transform3d"=w149:T10)  [unwired: 9 in]
  n48 = call <vilib>:"Transform3d_Create_Trans3dRot3d.vi"("Rotation3d"=w100, "Translation3d"=w101) -> ("Transform3d"=w99:T10)  [unwired: 9 in]
  n49 = call <vilib>:"Transform3d_Create_Trans3dRot3d.vi"("Rotation3d"=w108, "Translation3d"=w109) -> ("Transform3d"=w98:T10)  [unwired: 9 in]
  n50 = call <vilib>:"PhotonTrackedTarget_New.vi"("Pitch"=w242, "Yaw"=w247, "Fiducial Id"=w245, "Area"=w243, "Skew"=w244, "ObjDetectId"=0, "DetectedCorners"=w216, "DetectObjConf"=sgl 0.0, "BestCameraToTarget"=w199, "AltCameraToTarget"=w198, "MinAreaRectCorners"=w217, "Pose Ambiguity"=w246) -> ("TrackedTarget"=w97:T13)  [unwired: 3 in]
  n51 = call <vilib>:"PhotonTrackedTarget_New.vi"("Pitch"=w192, "Yaw"=w197, "Fiducial Id"=w195, "Area"=w193, "Skew"=w194, "ObjDetectId"=0, "DetectedCorners"=w166, "DetectObjConf"=sgl 0.0, "BestCameraToTarget"=w149, "AltCameraToTarget"=w148, "MinAreaRectCorners"=w167, "Pose Ambiguity"=w196) -> ("TrackedTarget"=w96:T13)  [unwired: 3 in]
  n52 = call <vilib>:"PhotonTrackedTarget_New.vi"("Pitch"=w142, "Yaw"=w147, "Fiducial Id"=w145, "Area"=w143, "Skew"=w144, "ObjDetectId"=0, "DetectedCorners"=w116, "DetectObjConf"=sgl 0.0, "BestCameraToTarget"=w99, "AltCameraToTarget"=w98, "MinAreaRectCorners"=w117, "Pose Ambiguity"=w146) -> ("TrackedTarget"=w95:T13)  [unwired: 3 in]
  n53 = call <vilib>:"Conv_Deg_Radians.vi"("Degress"=6.0) -> ("Radians"=w30:dbl)  [unwired: 10 in]
  n54 = call <vilib>:"Conv_Deg_Radians.vi"("Degress"=60.0) -> ("Radians"=w29:dbl)  [unwired: 10 in]
  n55 = call <vilib>:"Conv_Deg_Radians.vi"("Degress"=37.0) -> ("Radians"=w31:dbl)  [unwired: 10 in]
  n56 = call <vilib>:"Conv_Inches_Meters.vi"("INCH"=-11.0) -> ("Meters"=w32:dbl)  [unwired: 10 in]
  n57 = call <vilib>:"Conv_Inches_Meters.vi"("INCH"=-12.0) -> ("Meters"=w33:dbl)  [unwired: 10 in]
  n58 = call <vilib>:"Translation3d_Create.vi"("Z"=3.0 ("INCH"), "Y"=w32, "X"=w33) -> ("TRANSLATION3D"=w35:T3)  [unwired: 8 in]
  n59 = call <vilib>:"Rotation3d_Create_RollPitchYaw.vi"("Yaw"=w29, "Pitch"=w30, "Roll"=w31) -> ("Rotation3d"=w34:T4)  [unwired: 8 in]
  n60 = Build Array(w97, w96, w95) -> (w94:T13[])
  n61 = call <vilib>:"PhotonPipelineMetadata_New.vi"("TimeSinceLastPong"=w80, "SequenceID"=w79, "PublishTimestampMicros"=w78, "CaptureTimestampMicros"=w77) -> ("PhotonPipelineMetadata"=w76:T15)  [unwired: 7 in]
  n62 = call <vilib>:"PhotonPipelineResult_New.vi"("TrackedTargets"=w94, "Metadata"=w76) -> ("PhotonPipelineResult"=w93:T16)  [unwired: 9 in]
  n63 = call <vilib>:"Transform3d_Create_Trans3dRot3d.vi"("Rotation3d"=w34, "Translation3d"=w35) -> ("Transform3d"=w22:T10)  [unwired: 9 in]
  n64 = call <vilib>:"PhotonPipelineResult_SetTimeStampSecs.vi"("TimeStampSec"=10.5, "PhotonPipelineResult"=w93) -> ("Out PhotonPipelineResult"=w8:T16)  [unwired: 9 in]
  n65 = call <vilib>:"Rotation3d_Create_Default.vi"() -> ("ROTATION3D"=w6:T4)  [unwired: 11 in]
  n66 = call <vilib>:"PhotonPipelineResult_GetTimeStampSecs.vi"("PhotonPipelineResult"=w8) -> ("TimeStampSec"=w7:dbl)  [unwired: 10 in]
  n67 = flat-sequence {
    tunnel: w7 -> [w255]
    tunnel: w6 -> [w254]
    tunnel: [2.0 ("HighestAmbiguity")] -> w5
    frame #0 {
      n68 = call <vilib>:"PhotonPoseEstimator_AddHeadingData_Rotation3d.vi"("Heading"=w254, "TimeStamp"=w255) -> ()  [unwired: 10 in]
    }
    frame #1 {
    }
  }
  n69 = call <vilib>:"PhotonPoseEstimator_New.vi"("RobotToCamera"=w22, "Camera"=w42, "Strategy"=w41, "AprilTagFieldLayout"=w36) -> ("PhotonPoseEstimator"=w69:T1)  [unwired: 7 in]
  n70 = call <vilib>:"PhotonPoseEstimator_SetHighestAmbiguity.vi"("HighestAmbiguity"=w5, "PhotonPoseEstimator"=w69) -> ("out PhotonPoseEstimator"=w4:T1)  [unwired: 9 in]
  n71 = call <vilib>:"PhotonPoseEstimator_SetMultiTagFallbackStrategy.vi"("FallBack Strategy"=PhotonPoseStrategy_ENUM."PNP_DISTANCE_TRIG_SOLVE", "PhotonPoseEstimator"=w4) -> ("out PhotonPoseEstimator"=w3:T1)  [unwired: 9 in]
  n72 = call <vilib>:"PhotonPoseEstimator_Update_PipeResult.vi"("Has Results"=w37, "PipelineResult"=w8, "PhotonPoseEstimator"=w3) -> ("Pos Found"=→"Pos Found":bool, "PhotonEstimatedRobotPose"=w82:T12, "out PhotonPoseEstimator"=→"out PhotonPoseEstimator":T1)  [unwired: 6 in]
  "PhotonEstimatedRobotPose" <- w82
  n73 = call <vilib>:"PhotonPoseEstimator_PackConfig.vi"("RobotToCamera"=w22, "HighestAmbiguity"=w5, "PirmaryStrategy"=w41, "Camera"=w42) -> ("PoseEstimator_Configuration"=w39:T19)  [unwired: 7 in]
  n74 = call <vilib>:"PhotonPoseEstimator_Update_PnpDistanceTrigSolve.vi"("Has Results"=w37, "PipelineResult"=w8, "PhotonPoseEstimator"=w3) -> ("PhotonEstimatedRobotPose"=w40:T12)  [unwired: 6 in, 2 out]
  n75 = call <vilib>:"PhotonPoseEstimator_Execute_PnpDistanceTrigSolve.vi"("Configuration"=w39, "AprilTagFieldLayout"=w36, "PIpeline Has \nNew Results"=w37, "PipelineResult"=w8) -> ("PhotonEstimatedRobotPose"=w38:T12)  [unwired: 2 in, 5 out]
  n76 = Unbundle By Name(w82) -> ("EstimatedPose.Translation3d.X"=w85:dbl, "EstimatedPose.Translation3d.Y"=w84:dbl, "EstimatedPose.Translation3d.Z"=w83:dbl, "EstimatedPose.Rotation3d"=w21:T4)
  n77 = Unbundle By Name(w38) -> ("EstimatedPose.Translation3d.X"=w46:dbl, "EstimatedPose.Translation3d.Y"=w45:dbl, "EstimatedPose.Translation3d.Z"=w44:dbl)
  n78 = Unbundle By Name(w40) -> ("EstimatedPose.Translation3d.X"=w59:dbl, "EstimatedPose.Translation3d.Y"=w58:dbl, "EstimatedPose.Translation3d.Z"=w57:dbl)
  n79 = call <vilib>:"Rotation3d_GetXYZ.vi"("in Rotation3d"=w21) -> ("Z"=w9:dbl, "Y"=w10:dbl, "X"=w11:dbl)  [unwired: 8 in]
  n80 = call <vilib>:"Util_ApproxEquals.vi"("Tolerance"=0.01, "Value 2"=3.0, "Value 1"=w45) -> ("ApproxEquals"=w48:bool)  [unwired: 8 in]
  n81 = call <vilib>:"Util_ApproxEquals.vi"("Tolerance"=0.01, "Value 2"=1.0, "Value 1"=w46) -> ("ApproxEquals"=w53:bool)  [unwired: 8 in]
  n82 = call <vilib>:"Util_ApproxEquals.vi"("Tolerance"=0.01, "Value 2"=2.0, "Value 1"=w44) -> ("ApproxEquals"=w47:bool)  [unwired: 8 in]
  n83 = call <vilib>:"Util_ApproxEquals.vi"("Tolerance"=0.01, "Value 2"=4.42, "Value 1"=w84) -> ("ApproxEquals"=w87:bool)  [unwired: 8 in]
  n84 = call <vilib>:"Util_ApproxEquals.vi"("Tolerance"=0.01, "Value 2"=0.0, "Value 1"=w83) -> ("ApproxEquals"=w86:bool)  [unwired: 8 in]
  n85 = call <vilib>:"Util_ApproxEquals.vi"("Tolerance"=0.01, "Value 2"=7.3, "Value 1"=w85) -> ("ApproxEquals"=w250:bool)  [unwired: 8 in]
  n86 = call <vilib>:"Util_ApproxEquals.vi"("Tolerance"=0.01, "Value 2"=0.0, "Value 1"=w11) -> ("ApproxEquals"=w14:bool)  [unwired: 8 in]
  n87 = call <vilib>:"Util_ApproxEquals.vi"("Tolerance"=0.01, "Value 2"=0.0, "Value 1"=w10) -> ("ApproxEquals"=w13:bool)  [unwired: 8 in]
  n88 = call <vilib>:"Util_ApproxEquals.vi"("Tolerance"=0.01, "Value 2"=2.197, "Value 1"=w9) -> ("ApproxEquals"=w12:bool)  [unwired: 8 in]
  n89 = call <vilib>:"Util_ApproxEquals.vi"("Tolerance"=0.01, "Value 2"=3.0, "Value 1"=w58) -> ("ApproxEquals"=w61:bool)  [unwired: 8 in]
  n90 = call <vilib>:"Util_ApproxEquals.vi"("Tolerance"=0.01, "Value 2"=1.0, "Value 1"=w59) -> ("ApproxEquals"=w66:bool)  [unwired: 8 in]
  n91 = call <vilib>:"Util_ApproxEquals.vi"("Tolerance"=0.01, "Value 2"=2.0, "Value 1"=w57) -> ("ApproxEquals"=w60:bool)  [unwired: 8 in]
  n92 = Compound Arithmetic op=AND(w53, w48, w47) -> (w43:bool)
  "Test 2 Passed" <- w43
  n93 = Compound Arithmetic op=AND(w66, w61, w60) -> (w56:bool)
  "Test 1 Passed" <- w56
  n94 = Compound Arithmetic op=AND(w250, w87, w86, w14, w13, w12) -> (w248:bool)
  "Test 0 Passed" <- w248
  n95 = Compound Arithmetic op=AND(w248, w56, w43) -> (→"Test Passed":bool)
  "error out" <- "error in (no error)"
